vi "FPGA_SystemFPGA Ref Global.vi"() -> ()   [LabVIEW 2017]
uses:
  <vilib>/Rock Robotics/SystemInterfaces/System/FPGA_SystemFRC FPGA Ref.ctl
panel:
  out "FRC FPGA Status":errorcluster
  out "FRC FPGA Ref":T1
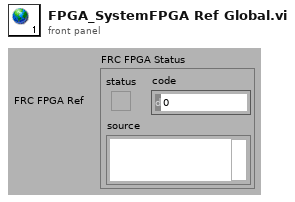
[diagram p1: front panel]
types:
  T1 = typedef "FPGA_SystemFRC FPGA Ref.ctl" = refnum<k20>
diagram:
